vi "Actor Core.vi"(8 "Error In":errorcluster, 11 "Core In":refnum<class "Core.lvclass">) -> (0 "Error Out":errorcluster, 3 "Actor Out":refnum<class "Actor.lvclass">)   [LabVIEW 2019, in "Core.lvlib" / "Core.lvclass"]
doc: "(<B>Filename</B>: Actor Framework.lvlib:Actor.lvclass:Actor Core.vi)\n\nReceives messages to the actor, reacts to them, and initiates any error handling that may shut the actor down.\n\nDescendant classes may override this VI to append parallel tasks for the actor to complete while it handles messages. Overrides use the Call Parent Method node."
uses:
  Core.lvclass
  C:/Projekty/_Wewnetrzne/PC_ActorFramework/07_Program/LABVIEW/02_Source/Modules/ModuleAbstract/ModuleAbstract.lvclass
  <vilib>/ActorFramework/Actor/Actor.lvclass
  SubModules/EventLog/EventLog.lvclass
  ModuleAbstract/ModuleAbstract.lvclass/ModuleAbstract.ctl
  Containers/ActorRefContainer/ActorRefContainer.lvclass/ActorRefContainer.ctl
  <vilib>/ActorFramework/Message Enqueuer/Message Enqueuer.lvclass/Message Enqueuer.ctl
  Containers/ActorRefContainer/Accessors/ActorRefContainer Read Logs.vi
  Containers/ActorRefContainer/Accessors/ActorRefContainer Read Modules.vi
  <vilib>/ActorFramework/Message Enqueuer/Enqueue.vi
  <vilib>/ActorFramework/Stop Msg/Stop Msg.lvclass
  C:/Program Files (x86)/National Instruments/LabVIEW 2019/vi.lib/ActorFramework/Message/Message.lvclass
  <vilib>/ActorFramework/Message Priority Queue/Priority Enqueue.vi
  <vilib>/ActorFramework/Message Enqueuer/Message Enqueuer.lvclass
  ModuleAbstract/ModuleAbstract.lvclass
  C:/Program Files (x86)/National Instruments/LabVIEW 2019/vi.lib/ActorFramework/Actor/Actor.lvclass
  C:/Projekty/_Wewnetrzne/PC_ActorFramework/07_Program/LABVIEW/02_Source/SubModules/LogsAbstract/LogsAbstract.lvclass
panel:
  in  "Stop":bool
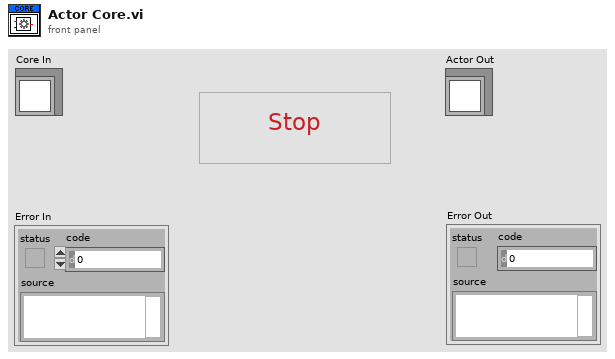
[diagram p1: front panel]
types:
  T1 = enum32{"Invalid", "Standard", "Closed", "Hidden", "Minimized", "Maximized"}
  T2 = cluster{"Core":cluster{"ModuleRef":refnum<class "Message Enqueuer.lvclass">, "UIRef":refnum<class "Message Enqueuer.lvclass">}}
  T3 = cluster{"EventLog":cluster{"ModRef":refnum<class "Message Enqueuer.lvclass">, "UIRef":refnum<class "Message Enqueuer.lvclass">}}
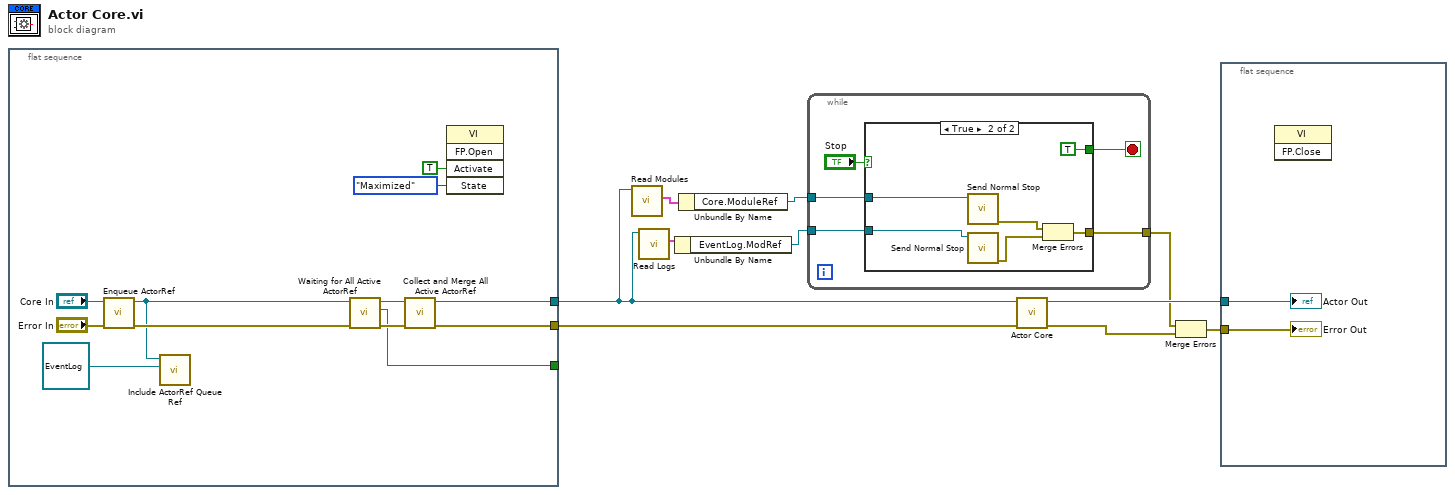
[diagram p0: block diagram]
diagram:
  n1 = flat-sequence {
    tunnel: [w16] -> w6
    tunnel: [w18] -> w5
    tunnel: [w15] -> _
    frame #0 {
      n2 = call-dynamic "Enqueue ActorRef.vi"("error in (no error)"="Error In", "Core in"="Core In") -> ("error out"=w13:errorcluster, "Core out"=w11:refnum<class "Core.lvclass">)  [unwired: 8 in]
      n3 = call "Include ActorRef Queue Ref.vi"("NestedModule In"=refnum<class "EventLog.lvclass"> refnum ("EventLog.lvlib:EventLog.lvclass"), "LaunchingModule"=w11) -> ()  [unwired: 8 in, 2 out]
      n4 = call "Waiting for All Active ActorRef.vi"("Error In"=w13, "Core In"=w11) -> ("Error Out"=w19:errorcluster, "Timeout"=w15:bool, "Core Out"=w20:refnum<class "Core.lvclass">)  [unwired: 7 in]
      n5 = call "Collect and Merge All Active ActorRef.vi"("Error In"=w19, "Core In"=w20) -> ("Error Out"=w16:errorcluster, "Core Out"=w18:refnum<class "Core.lvclass">)  [unwired: 8 in]
      n6 = invoke class="VI" method="FP.Open"("Activate"=TRUE ("Activate?"), "State"=T1."Maximized") -> ()  [unwired: 3 in, 5 out]
    }
  }
  n7 = call "Read Modules.vi"("ModuleAbstract in"=w5) -> ("Modules"=w2:T2)  [unwired: 8 in, 2 out]
  n8 = call "Read Logs.vi"("ModuleAbstract in"=w5) -> ("Logs"=w4:T3)  [unwired: 8 in, 2 out]
  n9 = Unbundle By Name(w4) -> ("EventLog.ModRef"=w3:refnum<class "Message Enqueuer.lvclass">)
  n10 = Unbundle By Name(w2) -> ("Core.ModuleRef"=w1:refnum<class "Message Enqueuer.lvclass">)
  n11 = while {
    tunnel: w1 -> [w26]
    tunnel: w3 -> [w24]
    tunnel: [w23] -> w7
    stop <- w25 stop-if-true
    n12 = case shown="True" "Stop" {
      tunnel: w26 -> [_ w33]
      tunnel: [_ TRUE] -> w25
      tunnel: w24 -> [_ w29]
      tunnel: [_ w30] -> w23
      frame False {
      }
      frame True {
        n13 = call <vilib>:"Send Normal Stop.vi"("Message Enqueuer"=w33) -> ("error out"=w31:errorcluster)  [unwired: 10 in]
        n14 = call <vilib>:"Send Normal Stop.vi"("Message Enqueuer"=w29) -> ("error out"=w28:errorcluster)  [unwired: 10 in]
        n15 = Merge Errors(w31, w28) -> (w30:errorcluster)
      }
    }
  }
  n16 = call-parent "Actor Core.vi"("error in"=w6, "Actor in"=w5) -> ("error out"=w8:errorcluster, "Actor out"=w10:refnum<class "Actor.lvclass">)  [unwired: 8 in]
  n17 = Merge Errors(w7, w8) -> (w9:errorcluster)
  n18 = flat-sequence {
    tunnel: w10 -> [w35]
    tunnel: w9 -> [w34]
    frame #0 {
      n19 = invoke class="VI" method="FP.Close"() -> ()  [unwired: 3 in, 3 out]
      "Error Out" <- w34
      "Actor Out" <- w35
    }
  }
